vi "Discover Nodes.vi"(8 "Error In":errorcluster, 11 "ICAN":refnum<class "ICAN.lvclass">) -> (0 "Error Out":errorcluster)   [LabVIEW 2024, in "CANopen Master.lvlib" / "Network Mangement.lvclass"]
uses:
  Network Mangement.lvclass
  HAL/HAL/Protocols/ICAN/ICAN.lvclass
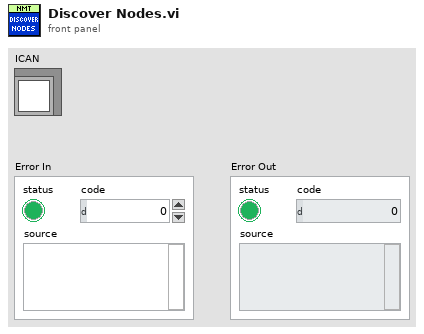
[diagram p1: front panel]
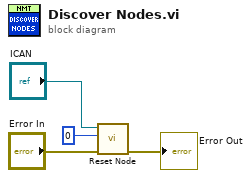
[diagram p0: block diagram]
diagram:
  n1 = call "Reset Node.vi"("Error In"="Error In", "Node-ID"=u8 0, "ICAN"="ICAN") -> ("Error Out"=→"Error Out":errorcluster)  [unwired: 8 in]
